vi "ma_sml_Next Good FFT Size.vi"(1 "FFT Size":i32) -> (0 "least bigger good size":i32)   [LabVIEW 2020, in "NI_MAPro.lvlib"]
uses:
  NI_MAPro.lvlib
panel:
  # "This VI returns the least bigger number contains prime factors all less than 13"
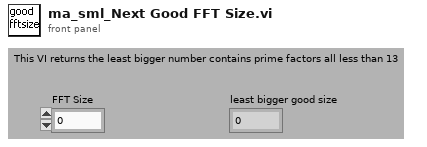
[diagram p1: front panel]
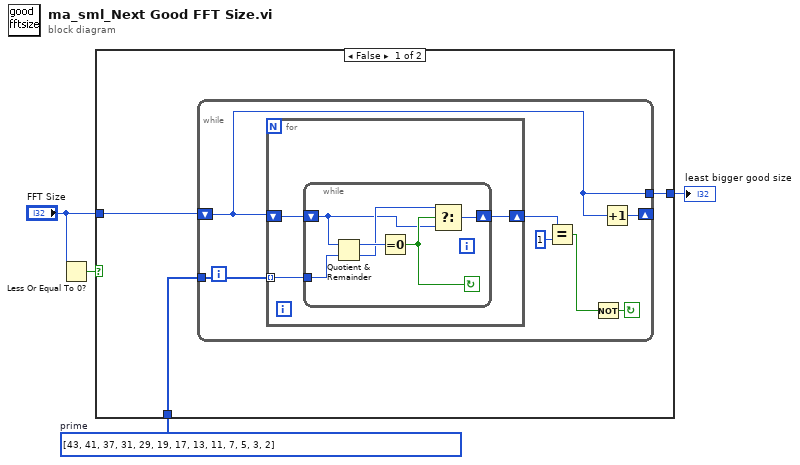
[diagram p0: block diagram]
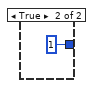
[diagram p2: hidden frame]
diagram:
  w1 = i32[] [43, 41, 37, 31, 29, 19, 17, 13, 11, 7, 5, 3, 2]  # prime
  n1 = Less Or Equal To 0?(x="FFT Size") -> (x <= 0?=w2:bool)
  n2 = case shown="False" w2 {
    tunnel: "FFT Size" -> [w7 _]
    tunnel: [w6 1 ("FFT Size")] -> w4
    tunnel: w1 -> [w5 _]
    frame False {
      n3 = while {
        tunnel: [w8] -> w6
        tunnel: w5 -> [w14]
        shift-left: w7 -> [w8]
        shift-right: [w9] -> _
        stop <- w11 continue-if-true
        n4 = for {
          tunnel: w14 -> [w17] mode=indexing
          shift-right: [w15] -> w10
          shift-left: w8 -> [w16]
          n5 = while {
            shift-left: w16 -> [w19]
            shift-right: [w22] -> w15
            tunnel: w17 -> [w18]
            stop <- w21 continue-if-true
            n6 = Quotient & Remainder(x=w19, y=w18) -> (x-y*floor(x/y)=w23:i32, floor(x/y)=w20:i32)
            n7 = Equal To 0?(x=w23) -> (x = 0?=w21:bool)
            n8 = Select(t=w20, s=w21, f=w19) -> (s? t:f=w22:i32)
          }
        }
        n9 = Equal?(x=w10, y=1) -> (x = y?=w12:bool)
        n10 = Not(x=w12) -> (.not. x?=w11:bool)
        n11 = Increment(x=w8) -> (x+1=w9:i32)
      }
    }
    frame True {
    }
  }
  "least bigger good size" <- w4
